vi "MBUS_TCP_Open.vi"(11 "ConnectionRefIn in":T1) -> (0 "error out":errorcluster, 3 "ConnectionRefIn out":T1)   [LabVIEW 2012, in "MBUS_Modbus.lvlib"]
uses:
  MBUS_Modbus.lvlib
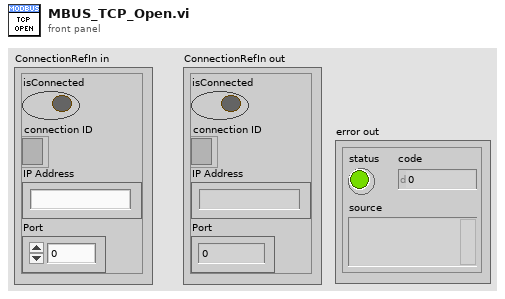
[diagram p1: front panel]
types:
  T1 = cluster{"isConnected":bool, "connection ID":refnum<k5>, "IP Address":string, "Port":dbl}
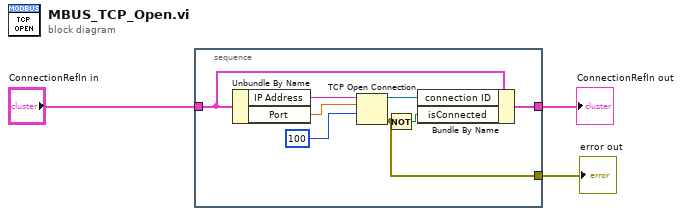
[diagram p0: block diagram]
diagram:
  n1 = stacked-sequence {
    tunnel: "ConnectionRefIn in" -> [w8]
    tunnel: [w5] -> w2
    tunnel: [w4] -> w1
    frame #0 {
      n2 = Unbundle By Name(w8) -> ("IP Address"=w11:string, "Port"=w10:dbl)
      n3 = TCP Open Connection(address=w11, remote port or service name=w10, timeout ms (60000)=100) -> (connection ID=w7:refnum<k5>, error out=w4:errorcluster)  [unwired: 2 in]
      n4 = Not(x=w4) -> (.not. x?=w6:bool)
      n5 = Bundle By Name(cluster=w8, "connection ID"=w7, "isConnected"=w6) -> (w5:T1)
    }
  }
  "ConnectionRefIn out" <- w2
  "error out" <- w1
